vi "linscale-elks.vi"() -> ()   [LabVIEW 2019]
panel:
  out "y":dbl[](array[numeric])
  out "XY Graph":cluster{"Y":dbl[], dbl[]}(graph)
  in  "b":dbl
  in  "a":dbl
  in  "X":dbl[](array[numeric])
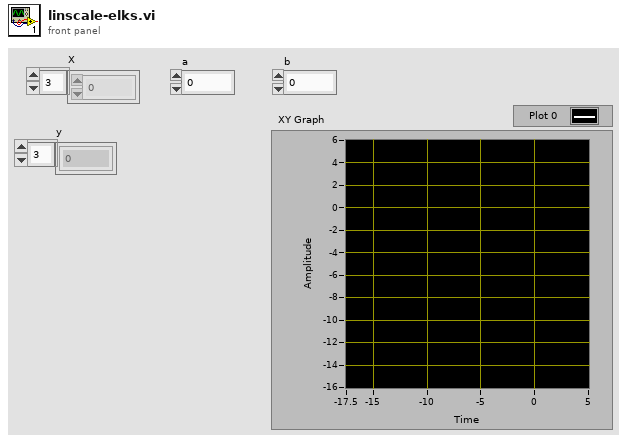
[diagram p1: front panel]
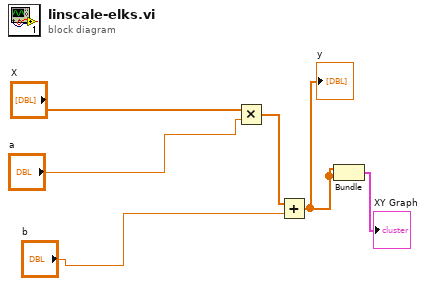
[diagram p0: block diagram]
diagram:
  n1 = Multiply(x="X", y="a") -> (x*y=w6:dbl[])
  n2 = Add(x=w6, y="b") -> (x+y=w2:dbl[])
  "y" <- w2
  n3 = Bundle(w2, w2) -> (→"XY Graph":cluster{dbl[], dbl[]})  [unwired: 1 in]
